vi "sendData.vi"(8 "error in (no error)":errorcluster, 11 "ILC in":refnum<class "ILC.lvclass">) -> (0 "error out":errorcluster, 3 "ILC out":refnum<class "ILC.lvclass">)   [LabVIEW 2013, in "ILCCommon.lvlib" / "ILC.lvclass"]
uses:
  <userlib>/Common/ILC/ILC/ILC.lvclass
  <userlib>/Common/ILC/ILC/ILC.lvclass/ILC.ctl
  <userlib>/Common/SerialProtocols/SerialCommunicator/SerialCommunicator.lvclass
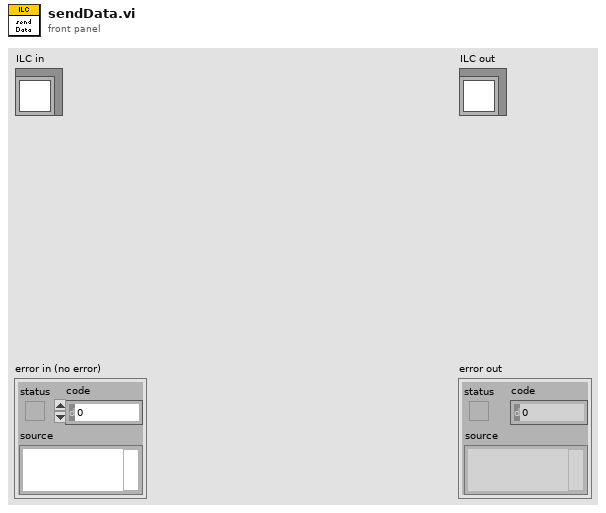
[diagram p1: front panel]
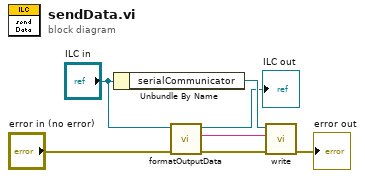
[diagram p0: block diagram]
diagram:
  n1 = Unbundle By Name("ILC in") -> ("serialCommunicator"=w6:refnum<class "SerialCommunicator.lvclass">)
  n2 = call <userlib>:"formatOutputData.vi"("error in (no error)"="error in (no error)", "ILC in"="ILC in") -> ("error out"=w4:errorcluster, "formattedOutputData"=w5:string, "ILC out"=→"ILC out":refnum<class "ILC.lvclass">)  [unwired: 7 in]
  n3 = call-dynamic "write.vi"("error in (no error)"=w4, "writeString"=w5, "SerialCommunicator in"=w6) -> ("error out"=→"error out":errorcluster)  [unwired: 7 in, 1 out]
